vi "Write Msg.Q.Ref.vi"(8 "error in (no error)":errorcluster, 10 "Msg.Q.Ref":T1, 11 "Messaging in":refnum<class "Messaging.lvclass">) -> (0 "error out":errorcluster, 3 "Messaging out":refnum<class "Messaging.lvclass">)   [LabVIEW 2023, in "Messaging.lvclass"]
uses:
  Messaging.lvclass
  Messaging.lvclass/Messaging.ctl
  Msg/Msg.Data.ctl
  Msg/Msg.Q.Ref.ctl
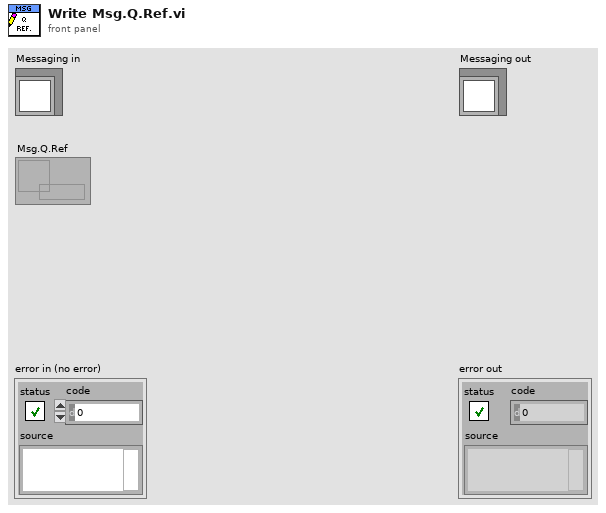
[diagram p1: front panel]
types:
  T1 = typedef "Msg.Q.Ref.ctl" = refnum<queue>
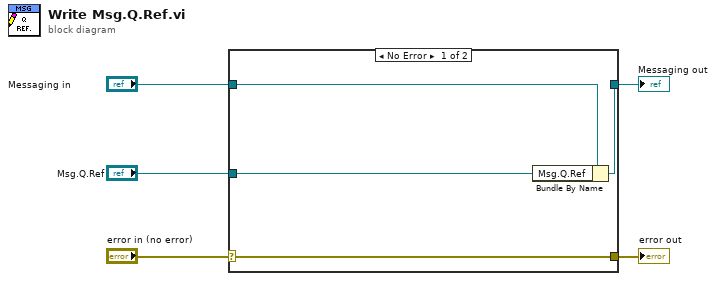
[diagram p0: block diagram]
diagram:
  n1 = case shown="No Error" "error in (no error)" {
    selector: "error in (no error)" -> [w9 w10]
    tunnel: [w9 w10] -> w4
    tunnel: [w7 w11] -> w2
    tunnel: "Messaging in" -> [w8 w11]
    tunnel: "Msg.Q.Ref" -> [w6 _]
    frame No Error {
      n2 = Bundle By Name(cluster=w8, "Msg.Q.Ref"=w6) -> (w7:refnum<class "Messaging.lvclass">)
    }
    frame Error {
    }
  }
  "error out" <- w4
  "Messaging out" <- w2
